vi "delWorkingPair.vi"(8 "Error (Input)":errorcluster, 11 "workingPair":i64) -> (0 "Error (Output)":errorcluster caption="Error(Output)")   [LabVIEW 2017]
doc: "delWorkingPair:\n * ---------------\n *\n * Destructor function to free allocated memory of a WorkingPair-struct.\n *\n * Parameters:\n * -----------\n * struct *WorkingPair:\n * Pointer of WorkingPair-struct.\n *\n * History:\n * --------\n * 01/06/2020, by Mirko Engelpracht:\n * First implementation.\n *\n */\nDLL_API void delWorkingPair(void *workingPair);\n\n\n/*\n * warning_struct:\n * ---------------\n *\n * Auxiliary function to throw warning if some struct (e.g. workingPair or\n * Adsorption) does not exist.\n *\n * Parameters:\n * -----------\n * const char *name_struct:\n * Name of struct that does not exist.\n * const char *name_function:\n * Name of function that does not exist.\n *\n * Returns:\n * --------\n * double:\n * Returns -1 to indicate error.\n *\n * History:\n * --------\n * 07/13/2021, by Jannik Driesel (supervised by Mirko Engelpracht):\n * First implementation."
uses:
  data/win32bit/libsorpPropLib.dll
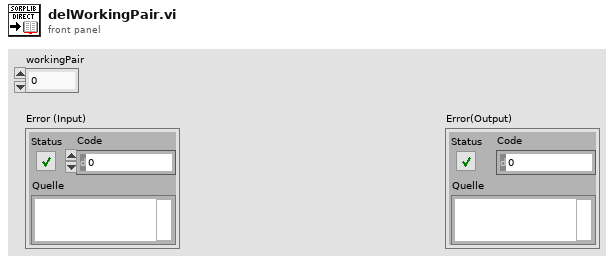
[diagram p1: front panel]
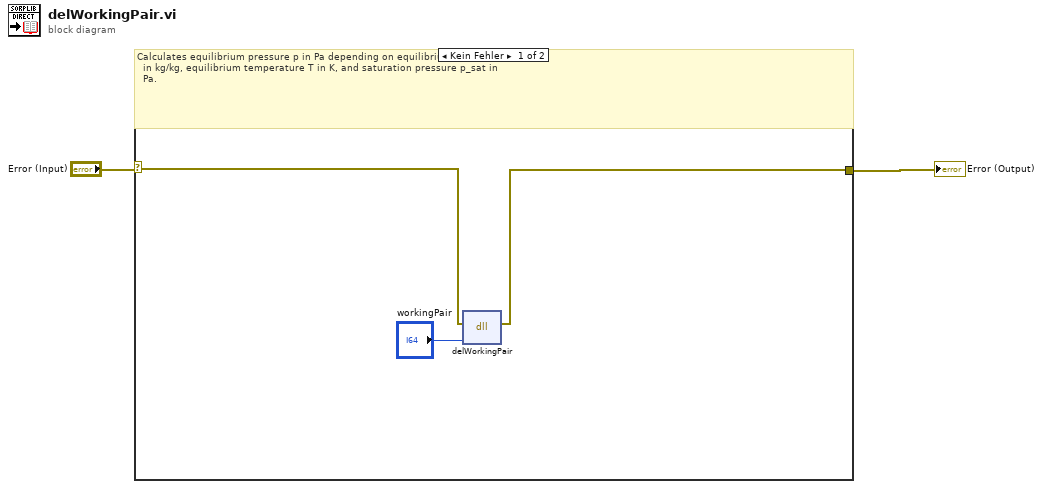
[diagram p0: block diagram]
diagram:
  n1 = case shown="Kein Fehler" "Error (Input)" {
    selector: "Error (Input)" -> [w5 w6]
    tunnel: [w4 w6] -> w1
    frame No Error {
      # "Calculates equilibrium pressure p in Pa depending on equilibrium loading w\n  in kg/kg, equilibrium temperature T in K, and saturation pressure p_sat in\n  Pa."
      n2 = dll-call lib="D:/Driesel/SorpLibLocal/LabVIEW_wrapper/data/win32bit/libsorpPropLib.dll" fn="delWorkingPair"(error in=w5, "workingPair"="workingPair") -> (error out=w4:errorcluster)  [unwired: 4 in, 1 out]
    }
    frame Error {
      # "Error - No calculations"
    }
  }
  "Error (Output)" <- w1
